vi "01.XX.16 Voltage output custom.vi"(0 "Write refnum in":refnum<file>, 2 "Step time":dbl, 3 "Sample Rate":dbl=1000.0, 4 "Number of Samples":i32=1000, 5 "Stop Custom In":refnum<vi>, 6 "Custom or file":bool, 7 "error in 2":errorcluster, 8 "array 2":dbl[][](array[numeric]), 10 "VS in":refnum<vi>, 11 "Sample Rate (actual)":refnum<vi>, 12 "VL in":refnum<vi>, 17 "Loop done logical":refnum<vi>, 18 "Stop":bool) -> (13 "error out 2":errorcluster, 14 "Write refnum out":refnum<file>, 19 "error out":errorcluster)   [LabVIEW 2017]
uses:
  <vilib>/DAQmx/write.llb/DAQmx Write (Analog 1D Wfm NChan NSamp).vi
  <vilib>/DAQmx/create/channels.llb/DAQmx Create Channel (AO-Voltage-Basic).vi
  <vilib>/DAQmx/configure/timing.llb/DAQmx Timing (Sample Clock).vi
  <vilib>/DAQmx/miscellaneous.llb/DAQmx Fill In Error Info.vi
  <resource>/objmgr/daqmx.rc
panel:
  out "Actual rate":dbl
  out "element":i32
  in  "VL":dbl
  in  "Vs":dbl
  out "logical OR":bool
  out "Numeric":i32
  out "appended array":dbl[][](array[numeric])
  # "© The Regents of the University of California, Davis campus, 2019. This material is available as open source for research and personal use under a Creative Commons Attribution-NonCommercial-NoDerivatives 4.0 International Public License (https://creativecommons.org/licenses/by-nc-nd/4.0/)."
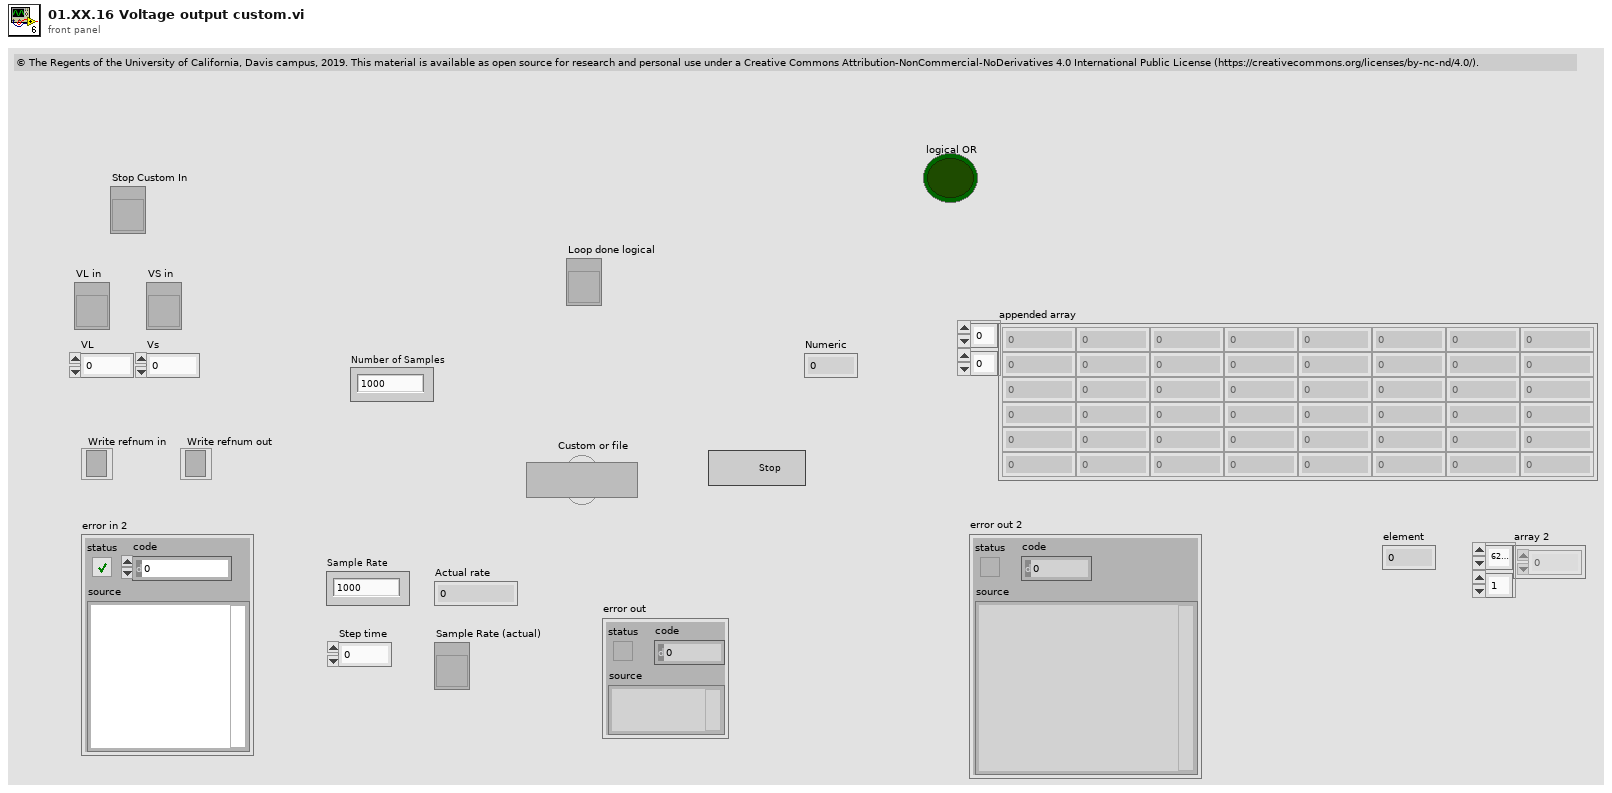
[diagram p1: front panel]
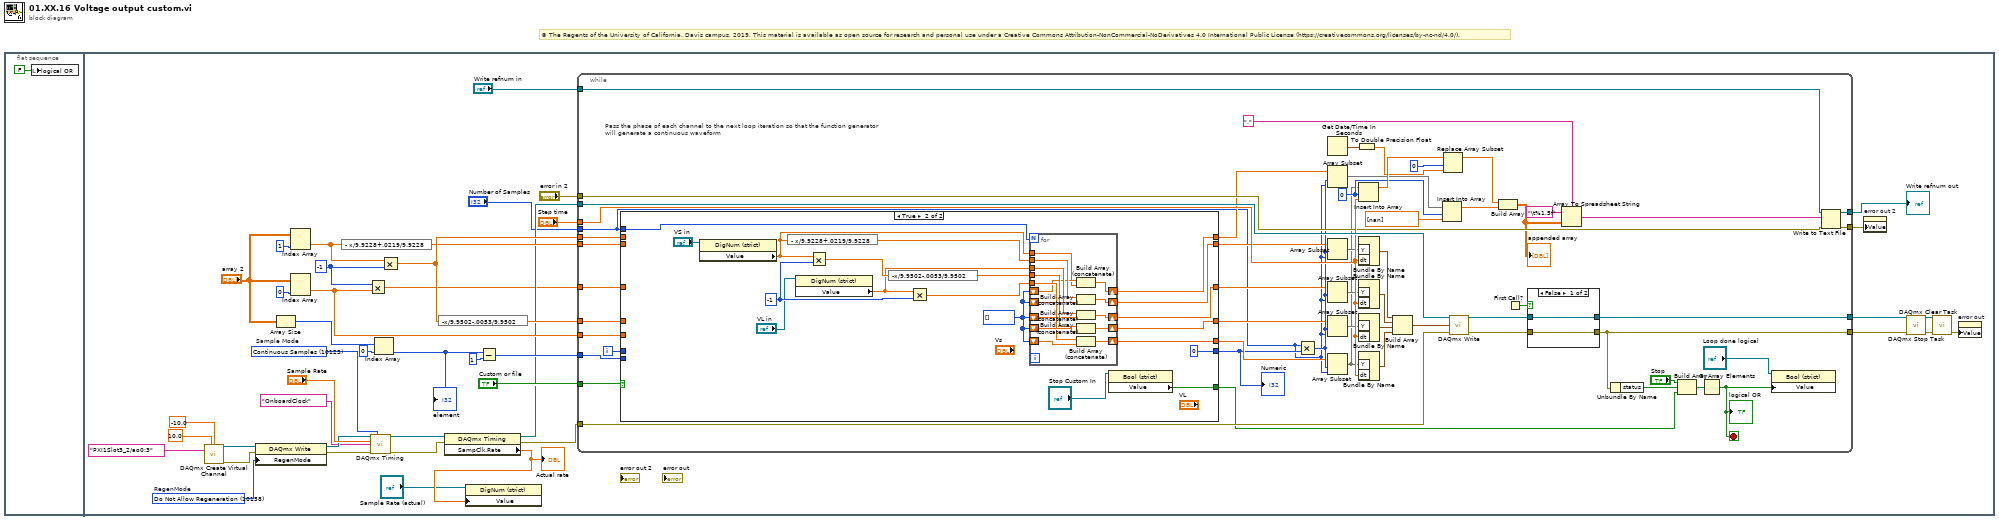
[diagram p0: block diagram]
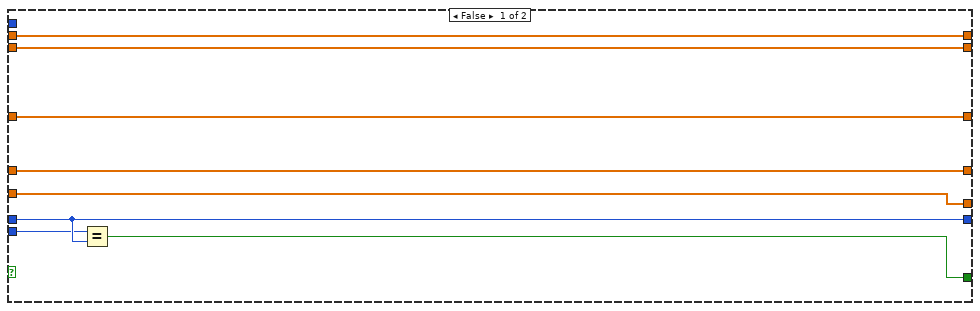
[diagram p2: hidden frame]
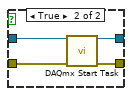
[diagram p3: hidden frame]
diagram:
  # "© The Regents of the University of California, Davis campus, 2019. This material is available as open source for research and personal use under a Creative Commons Attribution-NonCommercial-NoDerivatives 4.0 International Public License (https://creativecommons.org/licenses/by-nc-nd/4.0/)."
  n1 = flat-sequence {
    frame #0 {
      n2 = local write "logical OR"(FALSE ("logical OR")) -> ()
    }
    frame #1 {
      w24 = -1 ("disabled index (col)")
      w29 = 10123 items=["Finite Samples"=10178, "Continuous Samples"=10123, "Hardware Timed Single Point"=12522]  # Sample Mode
      w40 = 10158 items=["Allow Regeneration"=10097, "Do Not Allow Regeneration"=10158]  # RegenMode
      n3 = call-poly <vilib>:"DAQmx Create Virtual Channel.vi"("maximum value"=10.0 ("Max Voltage"), "minimum value"=-10.0 ("Max Voltage"), "physical channels"=tag "PXI1Slot3_2/ao0:3" ("Physical Channel(s)")) -> ("task out"=w42:refnum<k21>, "error out"=w41:errorcluster)  [unwired: 11 in]
      n4 = property class="DAQmx Write"(reference=w42, error in=w41, "RegenMode"=w40) -> (reference out=w38:refnum<k21>, error out=w39:errorcluster)
      n5 = Array Size(array="array 2") -> (size(s)=w20:i32[])
      n6 = Index Array(array="array 2", index (col)=1 ("disabled index (col)")) -> (element=w23:dbl[])  [unwired: 1 in]
      n7 = Index Array(array="array 2", index (col)=0 ("disabled index (col)")) -> (element=w9:dbl[])  [unwired: 1 in]
      n8 = expression code="- x/9.9228+.0219/9.9228"(w23) -> (w8:dbl[])
      n9 = Multiply(x=w24, y=w9) -> (x*y=w5:dbl[])
      n10 = call-poly <vilib>:"DAQmx Timing.vi"("task/channels in"=w38, "sample mode"=w29, "rate"="Sample Rate", "source"=tag "OnboardClock" ("Sample Clock Source"), "error in"=w39) -> ("task out"=w45:refnum<k21>, "error out"=w44:errorcluster)  [unwired: 9 in]
      n11 = Index Array(array=w20, index=0) -> (element=w18:i32)
      "element" <- w18
      n12 = Multiply(x=w23, y=w24) -> (x*y=w22:dbl[])
      n13 = expression code="-x/9.9502-.0053/9.9502"(w22) -> (w10:dbl[])
      n14 = property class="DAQmx Timing"(reference=w45, error in=w44) -> (reference out=w6:refnum<k21>, error out=w11:errorcluster, "SampClk.Rate"=w3:dbl)
      "Actual rate" <- w3
      n15 = property on="Property Node" class="DigNum (strict)"(reference="Sample Rate (actual)", "Value"=w3) -> ()  [unwired: 1 in, 2 out]
      n16 = Subtract(x=w18, y=1) -> (x-y=w16:i32)
      n17 = while {
        tunnel: w11 -> [w95]
        tunnel: w6 -> [w101]
        tunnel: [w100] -> w35
        tunnel: [w99] -> w34
        tunnel: "Write refnum in" -> [w98]
        tunnel: [w97] -> w15
        tunnel: [w96] -> w13
        tunnel: "error in 2" -> [w93]
        tunnel: w10 -> [w90]
        tunnel: w8 -> [w89]
        tunnel: w5 -> [w87]
        tunnel: w9 -> [w88]
        tunnel: "Step time" -> [w94]
        tunnel: w22 -> [w92]
        tunnel: w16 -> [w91]
        tunnel: "Custom or file" -> [w85]
        tunnel: "Number of Samples" -> [w46]
        i -> [w86]
        stop <- w84 stop-if-true
        w68 = 0 ("index (row)")
        # "Pass the phase of each channel to the next loop iteration so that the function generator will generate a continuous waveform"
        n18 = case shown="True" w85 {
          tunnel: w92 -> [w109 _]
          tunnel: [w109 w119] -> w54
          tunnel: w91 -> [w102 _]
          tunnel: w90 -> [w108 _]
          tunnel: [w108 w125] -> w53
          tunnel: w89 -> [w107 _]
          tunnel: [w107 w123] -> w52
          tunnel: [w106 w122] -> w51
          tunnel: w88 -> [w106 _]
          tunnel: w87 -> [w105 _]
          tunnel: [w105 w121] -> w50
          tunnel: w86 -> [w104 _]
          tunnel: [w104 0 ("y")] -> w49
          tunnel: w46 -> [_ w124]
          tunnel: [w103 w116] -> w48
          frame False {
            n19 = Equal?(x=w102, y=w104) -> (x = y?=w103:bool)
          }
          frame True {
            w120 = i32[] []
            w127 = -1 ("y")
            n20 = property on="Property Node" class="DigNum (strict)"(reference="VS in") -> ("Value"=w112:dbl)  [unwired: 1 in, 2 out]
            n21 = expression code="- x/9.9228+.0219/9.9228"(w112) -> (w128:dbl)
            n22 = property on="Property Node" class="DigNum (strict)"(reference="VL in") -> ("Value"=w111:dbl)  [unwired: 1 in, 2 out]
            n23 = Multiply(x=w112, y=w127) -> (x*y=w113:dbl)
            n24 = expression code="-x/9.9502-.0053/9.9502"(w113) -> (w126:dbl)
            n25 = Multiply(x=w111, y=w127) -> (x*y=w110:dbl)
            n26 = for {
              N: w124 -> [_]
              shift-right: [w143] -> w123
              shift-left: w120 -> [w142]
              tunnel: w128 -> [w141]
              tunnel: w126 -> [w139]
              shift-right: [w138] -> w125
              shift-left: w120 -> [w140]
              tunnel: w111 -> [w135]
              shift-right: [w136] -> w121
              shift-left: w120 -> [w137]
              tunnel: w110 -> [w133]
              shift-right: [w132] -> w122
              shift-left: w120 -> [w134]
              tunnel: w112 -> [w130]
              shift-right: [w129] -> w119
              shift-left: w120 -> [w131]
              n27 = Build Array (concatenate)(w131, w130) -> (w129:dbl[])
              n28 = Build Array (concatenate)(w141, w142) -> (w143:dbl[])
              n29 = Build Array (concatenate)(w135, w137) -> (w136:dbl[])
              n30 = Build Array (concatenate)(w139, w140) -> (w138:dbl[])
              n31 = Build Array (concatenate)(w133, w134) -> (w132:dbl[])
            }
            n32 = property on="Property Node" class="Bool (strict)"(reference="Stop Custom In") -> ("Value"=w116:bool)  [unwired: 1 in, 2 out]
          }
        }
        "Numeric" <- w49
        n33 = Multiply(x=w46, y=w49) -> (x*y=w64:i32)
        n34 = Get Date/Time In Seconds() -> (seconds since 1Jan1904=w83:timestamp)
        n35 = Array Subset(array=w54, index=w64, length=w46) -> (w63:dbl[])
        n36 = Array Subset(array=w52, index=w64, length=w46) -> (w76:dbl[])
        n37 = Array Subset(array=w50, index=w64, length=w46) -> (w75:dbl[])
        n38 = Array Subset(array=w53, index=w64, length=w46) -> (w74:dbl[])
        n39 = Array Subset(array=w51, index=w64, length=w46) -> (w60:dbl[])
        n40 = To Double Precision Float(number=w83) -> (double precision float=w59:dbl)
        n41 = Bundle By Name("Y"=w76, "dt"=w94) -> (w62:waveform(dbl))  [unwired: 1 in]
        n42 = Bundle By Name("Y"=w75, "dt"=w94) -> (w65:waveform(dbl))  [unwired: 1 in]
        n43 = Bundle By Name("Y"=w74, "dt"=w94) -> (w61:waveform(dbl))  [unwired: 1 in]
        n44 = Bundle By Name("Y"=w60, "dt"=w94) -> (w72:waveform(dbl))  [unwired: 1 in]
        n45 = Insert Into Array(array=w60, index=w68, new element=w94) -> (w70:dbl[])
        n46 = Build Array(w62, w65, w61, w72) -> (w73:waveform(dbl)[])
        n47 = Insert Into Array(array=w63, index=w68, new element=dbl[] [nan] ("new element/subarray")) -> (w69:dbl[])
        n48 = Replace Array Subset(array=w70, new element=w59, index=0) -> (w67:dbl[])
        n49 = call-poly <vilib>:"DAQmx Write.vi"("task/channels in"=w101, "data"=w73, "error in"=w95) -> ("task out"=w82:refnum<k21>, "error out"=w81:errorcluster)  [unwired: 10 in, 1 out]
        n50 = Build Array(w67, w69) -> (w66:dbl[][])
        "appended array" <- w66
        n51 = First Call?() -> (First Call?: T/F=w80:bool)
        n52 = case shown="False" w80 {
          tunnel: w82 -> [w144 w149]
          tunnel: w81 -> [w145 w148]
          tunnel: [w144 w147] -> w100
          tunnel: [w145 w146] -> w99
          frame False {
          }
          frame True {
            n53 = call <vilib>:"DAQmx Start Task.vi"("task/channels in"=w149, "error in"=w148) -> ("task out"=w147:refnum<k21>, "error out"=w146:errorcluster)  [unwired: 12 in]
          }
        }
        n54 = Array To Spreadsheet String(delimiter (Tab)=",", array=w66, 3:"\t%1.5f" ("format string")) -> (spreadsheet string=w78:string)
        n55 = Unbundle By Name(w99) -> ("status"=w56:bool)
        n56 = Build Array("Stop", w56, w48) -> (w55:bool[])
        n57 = Or Array Elements(Boolean array=w55) -> (logical OR=w84:bool)
        "logical OR" <- w84
        n58 = property on="Property Node" class="Bool (strict)"(reference="Loop done logical", "Value"=w84) -> ()  [unwired: 1 in, 2 out]
        n59 = Write to Text File(file (use dialog)=w98, text=w78, error in=w93) -> (refnum out=w97:refnum<file>, error out=w96:errorcluster)  [unwired: 1 in, 1 out]
      }
      "Write refnum out" <- w15
      n60 = property on="error out 2" class="Clust (strict)"("Value"=w13) -> ()  [unwired: 2 in, 2 out]
      n61 = call <vilib>:"DAQmx Stop Task.vi"("task/channels in"=w35, "error in"=w34) -> ("task out"=w37:refnum<k21>, "error out"=w36:errorcluster)  [unwired: 12 in]
      n62 = call <vilib>:"DAQmx Clear Task.vi"("task in"=w37, "error in"=w36) -> ("error out"=w12:errorcluster)  [unwired: 13 in]
      n63 = property on="error out" class="Clust (strict)"("Value"=w12) -> ()  [unwired: 2 in, 2 out]
    }
  }
